vi "R Peaks Coordinates.vi"(1 "2D Loc + Amp":dbl[][](array[numeric]) format="%#.2g", 2 "Locations":dbl[](array[numeric]), 3 "R-Wave Location (s)":dbl[](array[numeric])) -> (0 "R Peaks Coords":cluster{dbl[], dbl[]})   [LabVIEW 2018]
panel:
  out "X coord":dbl[](array[numeric])
  out "Y coord":dbl[](array[numeric])
  out "R index":dbl[](array[numeric])
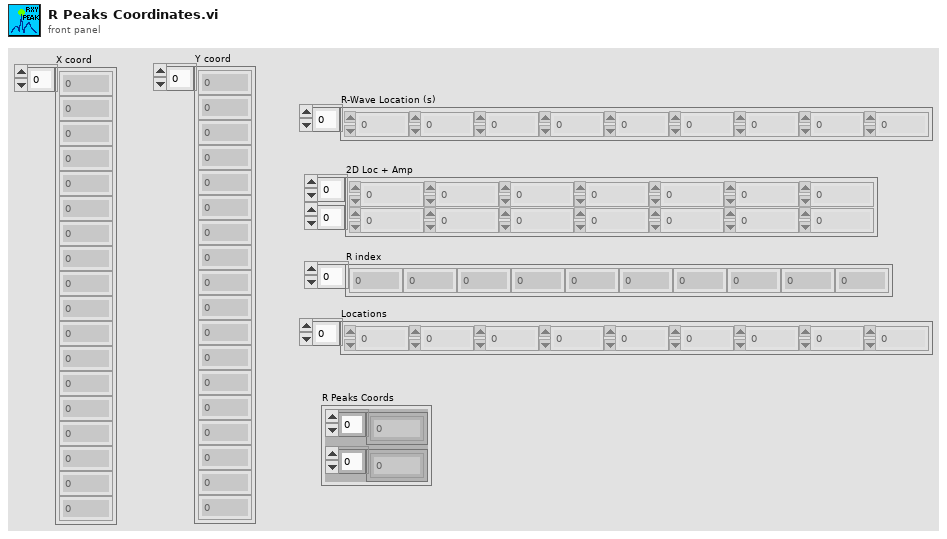
[diagram p1: front panel]
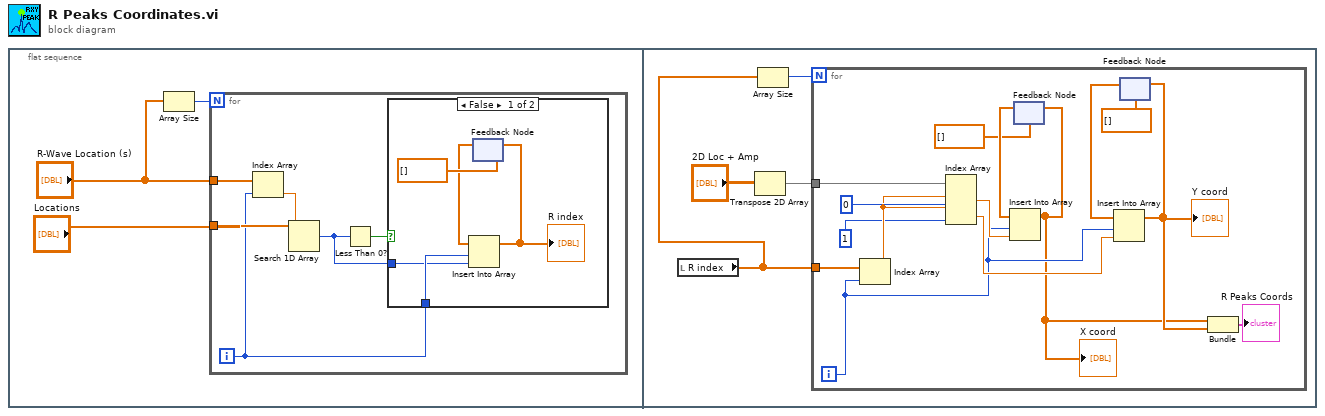
[diagram p0: block diagram]
diagram:
  n1 = flat-sequence {
    frame #0 {
      n2 = Array Size(array="R-Wave Location (s)") -> (size(s)=w3:i32)
      n3 = for {
        N: w3 -> [_]
        tunnel: "R-Wave Location (s)" -> [w8]
        tunnel: "Locations" -> [w9]
        i -> [w7]
        n4 = Index Array(array=w8, index=w7) -> (element=w6:dbl)
        n5 = Search 1D Array(1D array=w9, element=w6) -> (index of element=w5:i32)  [unwired: 1 in]
        n6 = Less Than 0?(x=w5) -> (x < 0?=w4:bool)
        n7 = case shown="False" w4 {
          tunnel: w7 -> [w11 _]
          tunnel: w5 -> [w10 _]
          frame False {
            n8 = feedback #1(dbl[] []) -> (w13:dbl[])
            n9 = Insert Into Array(array=w13, index=w11, new element=w10) -> (w12:dbl[])
            "R index" <- w12
            n10 = feedback-in #1(w12) -> ()
          }
          frame True {
          }
        }
      }
    }
    frame #1 {
      n11 = local read "R index"() -> (w17:dbl[])
      n12 = Transpose 2D Array(2D array="2D Loc + Amp") -> (transposed array=w16:dbl[][])
      n13 = Array Size(array=w17) -> (size(s)=w18:i32)
      n14 = for {
        N: w18 -> [_]
        tunnel: w16 -> [w33]
        tunnel: w17 -> [w29]
        i -> [w24]
        n15 = Index Array(array=w29, index=w24) -> (element=w27:dbl)
        n16 = Index Array(array=w33, index (row) #1=w27, index (col) #1=0 ("disabled index (col)"), index (row) #2=w27, index (col) #2=1 ("disabled index (col)")) -> (element #1=w31:dbl, element #2=w25:dbl)
        n17 = feedback #2(dbl[] []) -> (w32:dbl[])
        n18 = Insert Into Array(array=w32, index=w24, new element=w31) -> (w19:dbl[])
        "X coord" <- w19
        n19 = feedback-in #2(w19) -> ()
        n20 = feedback #3(dbl[] []) -> (w22:dbl[])
        n21 = Insert Into Array(array=w22, index=w24, new element=w25) -> (w21:dbl[])
        "Y coord" <- w21
        n22 = feedback-in #3(w21) -> ()
        n23 = Bundle(w19, w21) -> (→"R Peaks Coords":cluster{dbl[], dbl[]})  [unwired: 1 in]
      }
    }
  }
